vi "QD_Error_Logger.vi"(0 "State_and_Data_In":T1, 1 "Max_Queue_Size_In":i32=-1, 2 "Queue_Name_In":string, 5 "State_and_Data_N_In":T1[](array[typedef]), 7 "Time_Out_In_ms (-1)":i32, 11 "Error_In":errorcluster, 13 "Queue_Operation":T2=enum."Flush") -> (4 "State_and_Data_Out":T1, 15 "Error_Out":errorcluster)   [LabVIEW 2023]
doc: "Used to transfer data from one vi to another using queue."
uses:
  Controls/Queue_Operation_Select.ctl
  Controls/State_and_Data.ctl
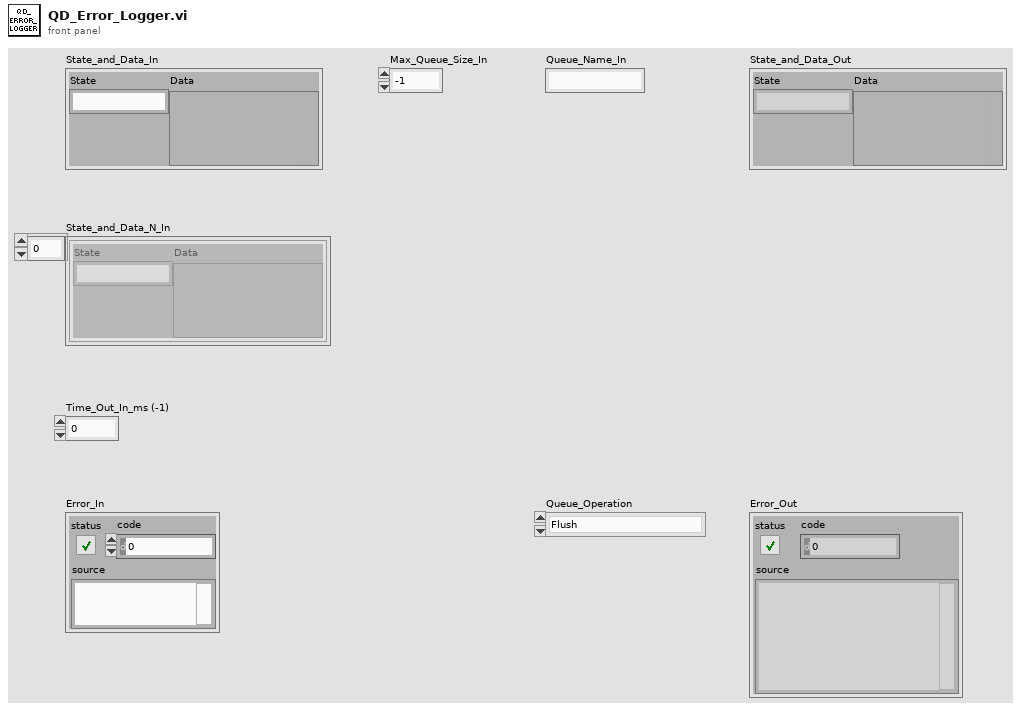
[diagram p1: front panel]
types:
  T1 = typedef "State_and_Data.ctl" = cluster{"State":string, "Data":variant}
  T2 = typedef "Queue_Operation_Select.ctl" = enum16{"Obtain_Queue", "Enqueue", "Enqueue_N", "Lossy_Enqueue", "Preview", "Queue_Status", "Release_Queue", "Dequeue", "Flush"}
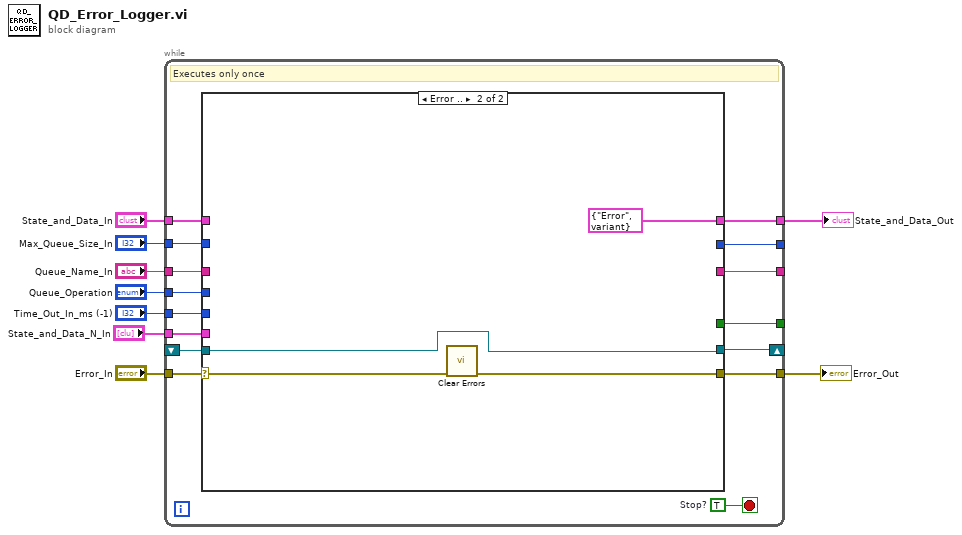
[diagram p0: block diagram]
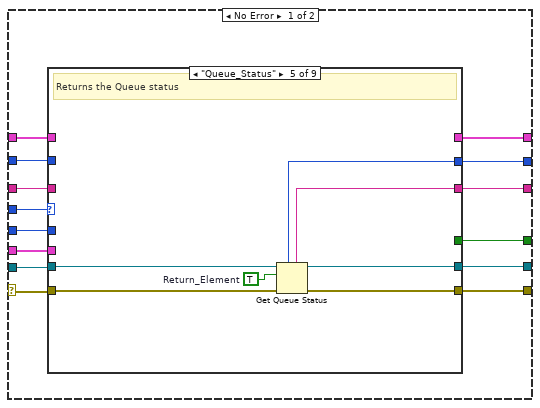
[diagram p2: hidden frame]
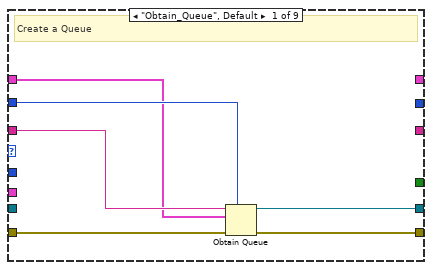
[diagram p3: hidden frame]
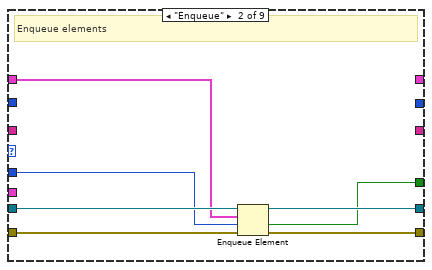
[diagram p4: hidden frame]
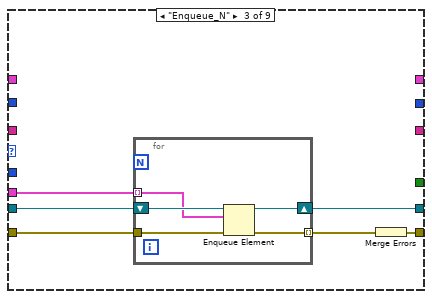
[diagram p5: hidden frame]
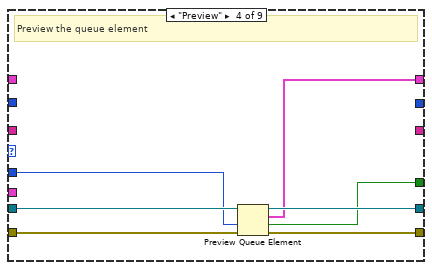
[diagram p6: hidden frame]
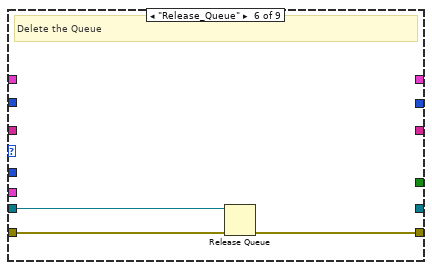
[diagram p7: hidden frame]
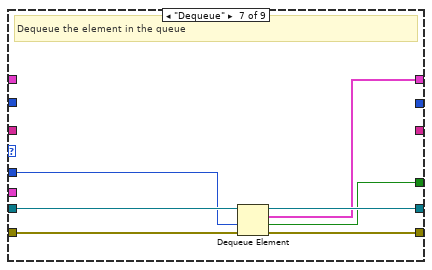
[diagram p8: hidden frame]
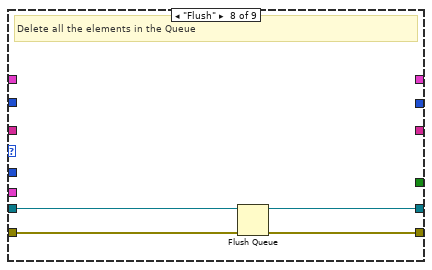
[diagram p9: hidden frame]
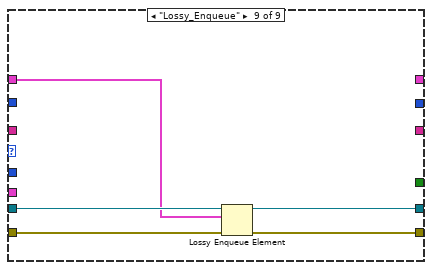
[diagram p10: hidden frame]
diagram:
  n1 = while {
    tunnel: "Max_Queue_Size_In" -> [w24]
    tunnel: "Time_Out_In_ms (-1)" -> [w21]
    tunnel: [w19] -> _
    tunnel: "Queue_Operation" -> [w16]
    shift-right: [w17] -> _
    shift-left: _ -> [w13]
    tunnel: "State_and_Data_In" -> [w22]
    tunnel: [w20] -> w2
    tunnel: "Queue_Name_In" -> [w15]
    tunnel: [w18] -> _
    tunnel: "Error_In" -> [w14]
    tunnel: [w23] -> w8
    tunnel: [w11] -> _
    tunnel: "State_and_Data_N_In" -> [w10]
    stop <- w12 stop-if-true
    w12 = TRUE  # Stop?
    # "Executes only once"
    n2 = case shown="Error .." w14 {
      selector: w14 -> [w28 w99]
      tunnel: w16 -> [w29 _]
      tunnel: w15 -> [w30 _]
      tunnel: w24 -> [w38 _]
      tunnel: [w37 w98] -> w17
      tunnel: [w36 w96] -> w23
      tunnel: w22 -> [w31 _]
      tunnel: w21 -> [w35 _]
      tunnel: [w34 T1 {"State"="Error", "Data"=variant} ("State_and_Data_In")] -> w20
      tunnel: [w33 _] -> w19
      tunnel: [w32 _] -> w18
      tunnel: w13 -> [w27 w98]
      tunnel: [w26 _] -> w11
      tunnel: w10 -> [w25 _]
      frame No Error {
        n3 = case shown="\"Queue_Status\"" w29 {
          tunnel: w28 -> [w44 w51 w57 w68 w75 w79 w85 w89 w94]
          tunnel: w30 -> [w42 _ _ _ _ _ _ _ _]
          tunnel: w38 -> [w41 _ _ _ _ _ _ _ _]
          tunnel: [w39 w47 w54 w67 w74 _ w84 w88 w93] -> w37
          tunnel: [w43 w50 w52 w66 w73 w78 w82 w87 w92] -> w36
          tunnel: w27 -> [_ w49 w55 w69 w76 w77 w86 w90 w95]
          tunnel: w31 -> [w40 w48 _ _ _ _ _ _ w91]
          tunnel: w35 -> [_ w46 _ w65 _ _ w81 _ _]
          tunnel: [_ _ _ w64 _ _ w83 _ _] -> w34
          tunnel: [_ _ _ _ w72 _ _ _ _] -> w33
          tunnel: [_ _ _ _ w71 _ _ _ _] -> w32
          tunnel: [_ w45 _ w63 _ _ w80 _ _] -> w26
          tunnel: w25 -> [_ _ w53 _ _ _ _ _ _]
          frame "Obtain_Queue", Default {
            # "Create a Queue"
            n4 = Obtain Queue(max queue size (-1, unlimited)=w41, name (unnamed)=w42, element data type=w40, error in (no error)=w44) -> (queue out=w39:refnum<queue>, error out=w43:errorcluster)  [unwired: 1 in, 1 out]
          }
          frame "Enqueue" {
            # "Enqueue elements"
            n5 = Enqueue Element(queue=w49, element=w48, timeout in ms (-1)=w46, error in (no error)=w51) -> (queue out=w47:refnum<queue>, timed out?=w45:bool, error out=w50:errorcluster)
          }
          frame "Enqueue_N" {
            n6 = for {
              tunnel: w53 -> [w58] mode=indexing
              tunnel: w57 -> [w62]
              tunnel: [w61] -> w56 mode=indexing
              shift-right: [w59] -> w54
              shift-left: w55 -> [w60]
              n7 = Enqueue Element(queue=w60, element=w58, error in (no error)=w62) -> (queue out=w59:refnum<queue>, error out=w61:errorcluster)  [unwired: 1 in, 1 out]
            }
            n8 = Merge Errors(w56) -> (w52:errorcluster)
          }
          frame "Preview" {
            # "Preview the queue element"
            n9 = Preview Queue Element(queue=w69, timeout in ms (-1)=w65, error in (no error)=w68) -> (queue out=w67:refnum<queue>, element=w64:T1, timed out?=w63:bool, error out=w66:errorcluster)
          }
          frame "Queue_Status" {
            w70 = TRUE  # Return_Element
            # "Returns the Queue status"
            n10 = Get Queue Status(queue=w76, return elements? (F)=w70, error in (no error)=w75) -> (queue out=w74:refnum<queue>, queue name=w71:string, max queue size=w72:i32, error out=w73:errorcluster)  [unwired: 4 out]
          }
          frame "Release_Queue" {
            # "Delete the Queue"
            n11 = Release Queue(queue=w77, error in (no error)=w79) -> (error out=w78:errorcluster)  [unwired: 1 in, 2 out]
          }
          frame "Dequeue" {
            # "Dequeue the element in the queue"
            n12 = Dequeue Element(queue=w86, timeout in ms (-1)=w81, error in (no error)=w85) -> (queue out=w84:refnum<queue>, element=w83:T1, timed out?=w80:bool, error out=w82:errorcluster)
          }
          frame "Flush" {
            # "Delete all the elements in the Queue"
            n13 = Flush Queue(queue=w90, error in (no error)=w89) -> (queue out=w88:refnum<queue>, error out=w87:errorcluster)  [unwired: 1 out]
          }
          frame "Lossy_Enqueue" {
            n14 = Lossy Enqueue Element(queue=w95, element=w91, error in (no error)=w94) -> (queue out=w93:refnum<queue>, error out=w92:errorcluster)  [unwired: 2 out]
          }
        }
      }
      frame Error {
        n15 = call <vilib>:"Clear Errors.vi"("error in (no error)"=w99) -> ("error out"=w96:errorcluster)  [unwired: 5 in, 1 out]
      }
    }
  }
  "Error_Out" <- w8
  "State_and_Data_Out" <- w2
